vi "Parallel VIs Launcher.vi"   [LabVIEW 2011]
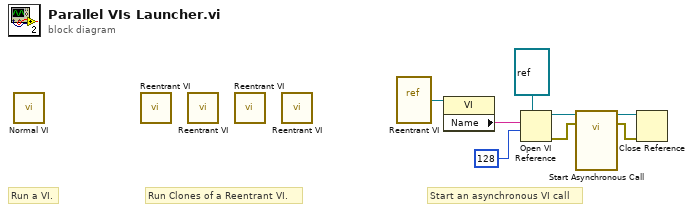
[diagram p0: block diagram]
diagram:
  # "Start an asynchronous VI call"
  # "Run a VI."
  # "Run Clones of a Reentrant VI."
  n1 = call "Normal VI.vi"() -> ()  [unwired: 12 in]
  n2 = call "Reentrant VI.vi"() -> ()  [unwired: 12 in]
  n3 = call "Reentrant VI.vi"() -> ()  [unwired: 12 in]
  n4 = call "Reentrant VI.vi"() -> ()  [unwired: 12 in]
  n5 = call "Reentrant VI.vi"() -> ()  [unwired: 12 in]
  n6 = vi-ref "Reentrant VI.vi"() -> (w2:refnum<vi>)
  n7 = property class="VI"(reference=w2) -> ("Name"=w1:string)  [unwired: 1 in, 2 out]
  n8 = Open VI Reference(type specifier VI Refnum (for type only)=refnum<vi> refnum, vi path=w1, options=128) -> (vi reference=w6:refnum<vi>, error out=w5:errorcluster)  [unwired: 3 in]
  n9 = call-by-ref "Start Asynchronous Call"(reference=w6, error in=w5) -> (reference out=w3:refnum<vi>, error out=w4:errorcluster)  [unwired: 12 in]
  n10 = Close Reference(reference=w3, error in (no error)=w4) -> ()  [unwired: 1 out]
